vi "solar_excel Worksheet Open.vi"(8 "error in (no error)":errorcluster, 10 "Sheet Name (STR) or Number (I32)":variant, 11 "Excel Workbook":T1) -> (0 "error out":errorcluster, 1 "Worksheet Index":i32, 2 "Worksheet Name":string, 3 "Excel Worksheet":T2)   [LabVIEW 2018]
doc: "This opens a Worksheet specified by 'Name' (String) or 'Number' (I32) and returns the Worksheet reference.\nNote: The first sheet is number '1'."
uses:
  solar_excel_ctl Worksheet.ctl
  solar_excel_ctl TSV.ctl
  solar_excel_ctl Workbook.ctl
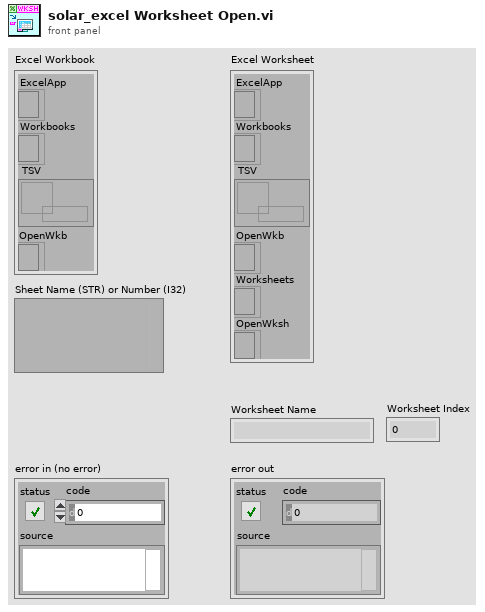
[diagram p1: front panel]
types:
  T1 = typedef "solar_excel_ctl Workbook.ctl" = cluster{"ExcelApp":refnum<k7>, "Workbooks":refnum<k7>, "TSV":refnum<queue>, "OpenWkb":refnum<k7>}
  T2 = typedef "solar_excel_ctl Worksheet.ctl" = cluster{"ExcelApp":refnum<k7>, "Workbooks":refnum<k7>, "TSV":refnum<queue>, "OpenWkb":refnum<k7>, "Worksheets":refnum<k7>, "OpenWksh":refnum<k7>}
  T3 = typedef "solar_excel_ctl TSV.ctl" = cluster{"Path":path, "Dirty":bool, "ActiveSheet":u8, "Worksheets":string[], "Worksheet Cells":cluster{"Cells":string[][]}[]}
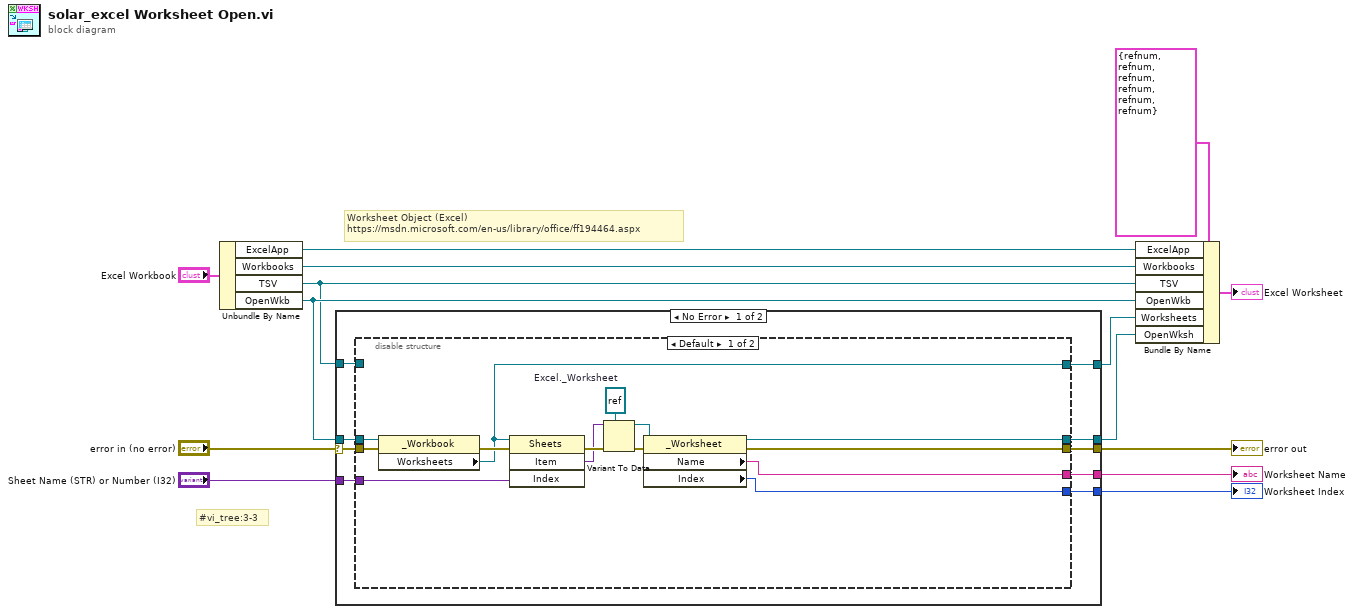
[diagram p0: block diagram]
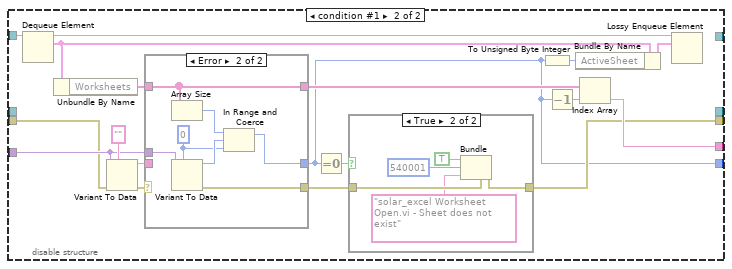
[diagram p2: hidden frame]
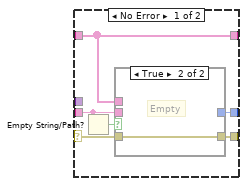
[diagram p4: hidden frame]
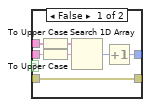
[diagram p5: hidden frame]
diagram:
  # "#vi_tree:3-3"
  # "Worksheet Object (Excel)\nhttps://msdn.microsoft.com/en-us/library/office/ff194464.aspx"
  n1 = Unbundle By Name("Excel Workbook") -> ("ExcelApp"=w10:refnum<k7>, "Workbooks"=w9:refnum<k7>, "TSV"=w1:refnum<queue>, "OpenWkb"=w8:refnum<k7>)
  n2 = case shown="No Error" "error in (no error)" {
    selector: "error in (no error)" -> [w23 w83]
    tunnel: [w19 w83] -> w14
    tunnel: w8 -> [w22 _]
    tunnel: [w21 _] -> w5
    tunnel: "Sheet Name (STR) or Number (I32)" -> [w20 _]
    tunnel: [w18 _] -> w4
    tunnel: [w17 _] -> w3
    tunnel: [w16 _] -> w2
    tunnel: w1 -> [w15 _]
    frame No Error {
      n3 = disable-structure shown="Default" {
        disable-tunnel: w23 -> [w37 w47]
        disable-tunnel: w22 -> [w34 _]
        disable-tunnel: [w33 _] -> w21
        disable-tunnel: w20 -> [w30 w48]
        disable-tunnel: [w28 w40] -> w19
        disable-tunnel: [w26 _] -> w18
        disable-tunnel: [w25 w43] -> w17
        disable-tunnel: [w24 w38] -> w16
        disable-tunnel: w15 -> [_ w55]
        frame condition #0 (active) {
          w29 = refnum<k7> refnum  # Excel._Worksheet
          n4 = property class="_Workbook"(reference=w34, error in=w37) -> (error out=w35:errorcluster, "Worksheets"=w33:refnum<k7>)  [unwired: 1 out]
          n5 = invoke class="Sheets" method="Item"(reference=w33, error in=w35, "Index"=w30) -> (error out=w36:errorcluster, "Item"=w31:variant)  [unwired: 1 in, 2 out]
          n6 = Variant To Data(error in=w36, type=w29, Variant=w31) -> (data=w27:refnum<k7>, error out=w32:errorcluster)
          n7 = property class="_Worksheet"(reference=w27, error in=w32) -> (reference out=w26:refnum<k7>, error out=w28:errorcluster, "Name"=w25:string, "Index"=w24:i32)
        }
        frame condition #1 {
          n8 = Dequeue Element(queue=w55) -> (queue out=w54:refnum<queue>, element=w52:T3)  [unwired: 2 in, 2 out]
          n9 = Unbundle By Name(w52) -> ("Worksheets"=w46:string[])
          n10 = Variant To Data(error in=w47, type="", Variant=w48) -> (data=w49:string, error out=w50:errorcluster)
          n11 = case shown="Error" w50 {
            selector: w50 -> [w64 _]
            tunnel: w49 -> [w63 _]
            tunnel: w48 -> [_ w82]
            tunnel: [w65 w81] -> w39
            tunnel: w46 -> [w66 w79]
            tunnel: [w67 w77] -> w38
            tunnel: [w66 w79] -> w42
            frame No Error {
              n12 = Empty String/Path?(string/path=w63) -> (empty?=w62:bool)
              n13 = case shown="True" w62 {
                tunnel: w63 -> [w73 _]
                tunnel: [w71 _] -> w67
                tunnel: w66 -> [w69 _]
                tunnel: [w68 w75] -> w65
                tunnel: w64 -> [w68 w75]
                frame False {
                  n14 = To Upper Case(1:w69) -> (0:w74:string[])
                  n15 = To Upper Case(1:w73) -> (0:w72:string)
                  n16 = Search 1D Array(1D array=w74, element=w72) -> (index of element=w70:i32)  [unwired: 1 in]
                  n17 = Increment(x=w70) -> (x+1=w71:i32)
                }
                frame True {
                  # "Empty"
                }
              }
            }
            frame Error {
              w76 = 0
              n18 = Array Size(array=w79) -> (size(s)=w78:i32)
              n19 = Variant To Data(type=w76, Variant=w82) -> (data=w80:i32, error out=w81:errorcluster)  [unwired: 1 in]
              n20 = In Range and Coerce(upper limit=w78, x=w80, lower limit=w76) -> (coerced(x)=w77:i32)  [unwired: 1 out]
            }
          }
          n21 = Equal To 0?(x=w38) -> (x = 0?=w41:bool)
          n22 = case shown="True" w41 {
            tunnel: [w56 w60] -> w40
            tunnel: w39 -> [w56 w61]
            frame False {
            }
            frame True {
              n23 = Bundle(cluster=w61, "status"=TRUE ("show call chain? (False)"), "code"=540001 ("error code (0)"), "source"="solar_excel Worksheet Open.vi - Sheet does not exist") -> (w60:errorcluster)
            }
          }
          n24 = To Unsigned Byte Integer(number=w38) -> (unsigned 8bit integer=w45:u8)
          n25 = Decrement(x=w38) -> (x-1=w44:i32)
          n26 = Bundle By Name(cluster=w52, "ActiveSheet"=w45) -> (w53:T3)
          n27 = Index Array(array=w42, index=w44) -> (element=w43:string)
          n28 = Lossy Enqueue Element(queue=w54, element=w53) -> ()  [unwired: 1 in, 4 out]
        }
      }
    }
    frame Error {
    }
  }
  "error out" <- w14
  "Worksheet Name" <- w3
  "Worksheet Index" <- w2
  n29 = Bundle By Name(cluster=T2 {"ExcelApp"=refnum, "Workbooks"=refnum, "TSV"=refnum, "OpenWkb"=refnum, "Worksheets"=refnum, "OpenWksh"=refnum} ("Excel Worksheet 2"), "ExcelApp"=w10, "Workbooks"=w9, "TSV"=w1, "OpenWkb"=w8, "Worksheets"=w5, "OpenWksh"=w4) -> (→"Excel Worksheet":T2)
